vi "get_translation_request.vi"(8 "error in (no error)":errorcluster, 11 "GenericStage.lvclass in":refnum<class "GenericStage.lvclass">) -> (0 "error out":errorcluster, 2 "translation request":T1, 3 "GenericStage.lvclass out":refnum<class "GenericStage.lvclass">)   [LabVIEW 2010, in "GenericStage.lvclass"]
uses:
  GenericStage.lvclass
  translation_request.ctl
  common/classes/SpaceVector/SpaceVector/SpaceVector.lvclass
  translation_mode_enum.ctl
  GenericStage.lvclass/GenericStage.ctl
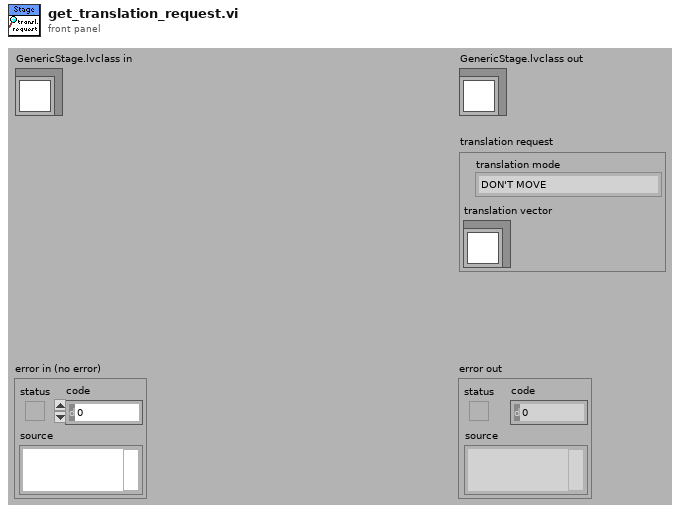
[diagram p1: front panel]
types:
  T1 = typedef "GenericStage.lvclass/translation_request.ctl" = cluster{"translation mode":T2, "translation vector":refnum<class "SpaceVector.lvclass">}
  T2 = typedef "GenericStage.lvclass/translation_mode_enum.ctl" = enum16{"DON'T MOVE", "relative", "absolute"}
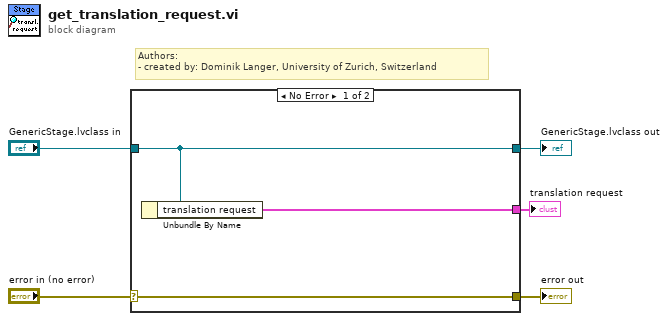
[diagram p0: block diagram]
diagram:
  # "Authors: \n- created by: Dominik Langer, University of Zurich, Switzerland"
  n1 = case shown="No Error" "error in (no error)" {
    selector: "error in (no error)" -> [w8 w9]
    tunnel: [w8 w9] -> w4
    tunnel: [w7 w10] -> w2
    tunnel: "GenericStage.lvclass in" -> [w7 w10]
    tunnel: [w6 _] -> w1
    frame No Error {
      n2 = Unbundle By Name(w7) -> ("translation request"=w6:T1)
    }
    frame Error {
    }
  }
  "error out" <- w4
  "GenericStage.lvclass out" <- w2
  "translation request" <- w1
